vi "Mutate Channel Group Commands.vi"(8 "error in":errorcluster, 11 "device in":T1 format="%.0x") -> (0 "error out":errorcluster, 3 "device out":T1 format="%.0x")   [LabVIEW 2027, in "Embedded Data Logger System Explorer.lvlib"]
uses:
  Embedded Data Logger System Explorer.lvlib
  <vilib>/NI VeriStand/Custom Device API/Custom Device Item Ref.ctl
  Shared/Constants.vi
  <vilib>/NI VeriStand/Custom Device Tools/Custom Device Utility Library/NI VeriStand - Search for All Items by GUID.vi
  <vilib>/NI VeriStand/Custom Device Tools/Custom Device Utility Library/NI VeriStand - Search for Item by GUID.vi
  <vilib>/NI VeriStand/Custom Device API/Get Item Property (I32).vi
  <vilib>/NI VeriStand/Custom Device Tools/Custom Device Utility Library/Custom Device Utility Library.lvlib
  Shared/Embedded Data Logger Shared.lvlib
  Scripting/Embedded Data Logger Scripting.lvlib
  <vilib>/NI VeriStand/Custom Device API/Custom Device API.lvlib
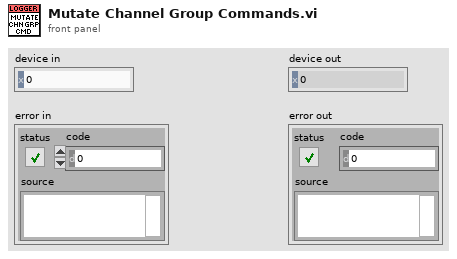
[diagram p1: front panel]
types:
  T1 = typedef "Custom Device API.lvlib/Custom Device Item Ref.ctl" = u64
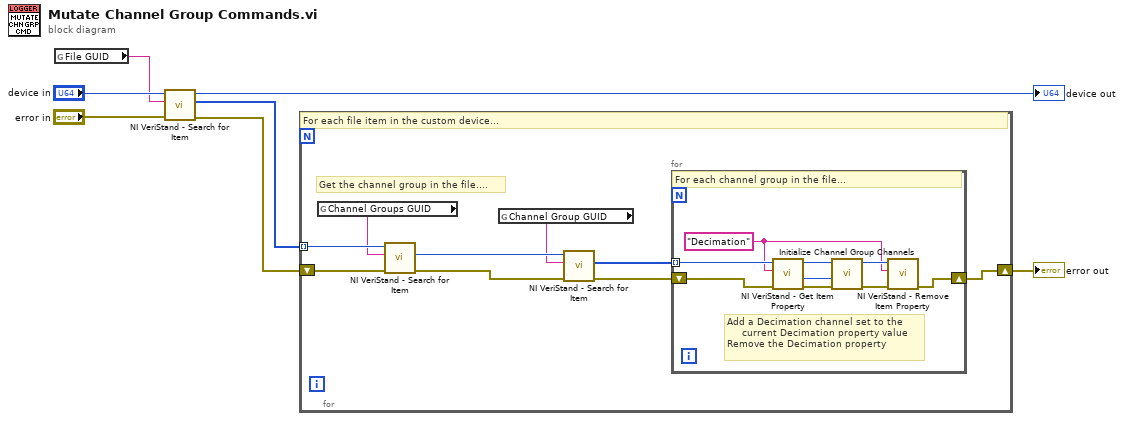
[diagram p0: block diagram]
diagram:
  n1 = global read "Constants.vi" "File GUID"() -> (w2:string)
  n2 = call-poly <vilib>:"NI VeriStand - Search for Item.vi"("error in"="error in", "Item GUID"=w2, "Section Ref in"="device in") -> ("error out"=w6:errorcluster, "Item Refs"=w7:T1[], "Section Ref out"=→"device out":T1)  [unwired: 1 in, 5 out]
  n3 = for {
    shift-right: [w12] -> w1
    shift-left: w6 -> [w14]
    tunnel: w7 -> [w16] mode=indexing
    # "Get the channel group in the file...."
    # "For each file item in the custom device..."
    n4 = global read "Constants.vi" "Channel Groups GUID"() -> (w11:string)
    n5 = call-poly <vilib>:"NI VeriStand - Search for Item.vi"("error in"=w14, "Item GUID"=w11, "Section Ref in"=w16) -> ("error out"=w13:errorcluster, "Item Ref"=w15:T1)  [unwired: 7 out]
    n6 = global read "Constants.vi" "Channel Group GUID"() -> (w10:string)
    n7 = call-poly <vilib>:"NI VeriStand - Search for Item.vi"("error in"=w13, "Item GUID"=w10, "Section Ref in"=w15) -> ("error out"=w8:errorcluster, "Item Refs"=w9:T1[])  [unwired: 1 in, 6 out]
    n8 = for {
      tunnel: w9 -> [w23] mode=indexing
      shift-right: [w17] -> w12
      shift-left: w8 -> [w21]
      w18 = "Decimation" ("Property Name")
      # "Add a Decimation channel set to the \n     current Decimation property value\nRemove the Decimation property"
      # "For each channel group in the file..."
      n9 = call-poly <vilib>:"NI VeriStand - Get Item Property.vi"("error in (no error)"=w21, "Property Name"=w18, "Item Ref in"=w23) -> ("error out"=w22:errorcluster, "Value"=w24:i32, "Item Ref out"=w25:T1)  [unwired: 1 in, 5 out]
      n10 = call "Initialize Channel Group Channels.vi"("error in"=w22, "default decimation value"=w24, "channel group reference in"=w25) -> ("error out"=w20:errorcluster, "channel group reference out"=w19:T1)  [unwired: 7 in]
      n11 = call <vilib>:"NI VeriStand - Remove Item Property.vi"("error in (no error)"=w20, "Property Name"=w18, "Item Ref in"=w19) -> ("error out"=w17:errorcluster)  [unwired: 6 in, 2 out]
    }
  }
  "error out" <- w1
